vi "DataTreeCtrl signalToIonData.vi"(8 "error in (no error)":errorcluster, 10 "signalData":waveform(sgl), 11 "DataTreeCtrl in":refnum<class "DataTreeCtrl.lvclass">) -> (0 "error out":errorcluster, 2 "ionSigInfo":T1, 3 "DataTreeCtrl out":refnum<class "DataTreeCtrl.lvclass">, 5 "plotName":string)   [LabVIEW 2018, in "DataTreeCtrl.lvclass"]
uses:
  DataTreeCtrl.lvclass
  DataTreeCtrl.lvclass/DataTreeCtrl.ctl
  PublicSubVI/Class/Sig2MS/Sig2MS.lvclass
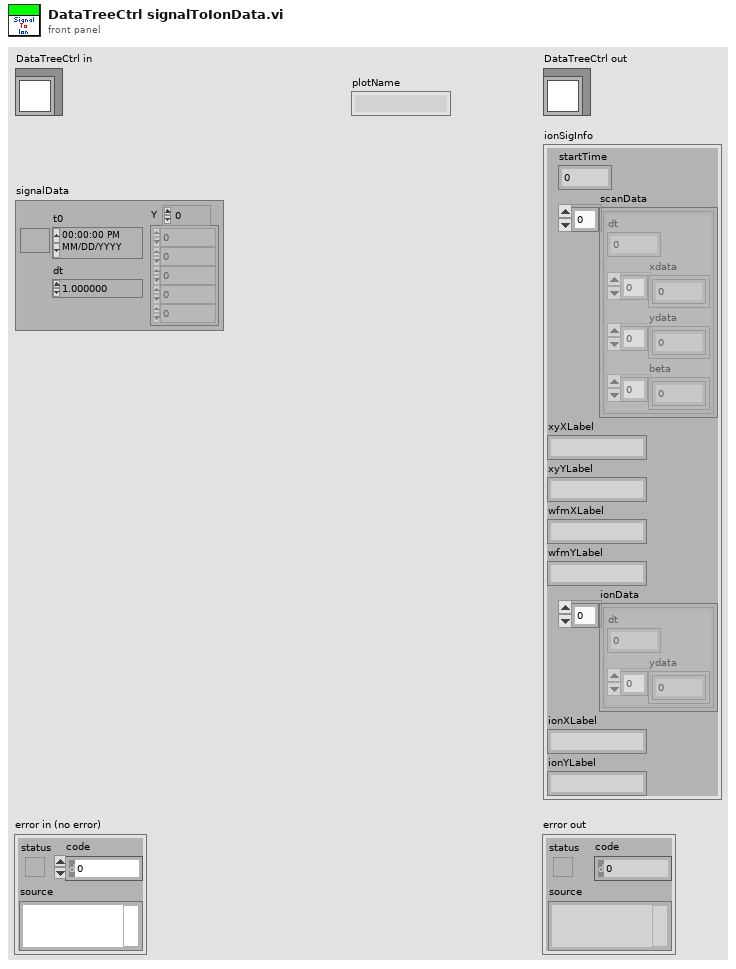
[diagram p1: front panel]
types:
  T1 = cluster{"startTime":dbl, "scanData":cluster{"dt":dbl, "xdata":dbl[], "ydata":sgl[], "beta":dbl[]}[], "xyXLabel":string, "xyYLabel":string, "wfmXLabel":string, "wfmYLabel":string, "ionData":cluster{"dt":dbl, "ydata":sgl[]}[], "ionXLabel":string, "ionYLabel":string}
  T2 = enum16{"init", "loadScript", "newScript", "runScript", "close"}
  T3 = cluster{"startTime":dbl, "scanSig":cluster{"priDt":dbl, "priXData":dbl[], "priYData":sgl[], "beta":dbl[]}[], "ionSig":cluster{"secDt":dbl, "secYData":sgl[]}[]}
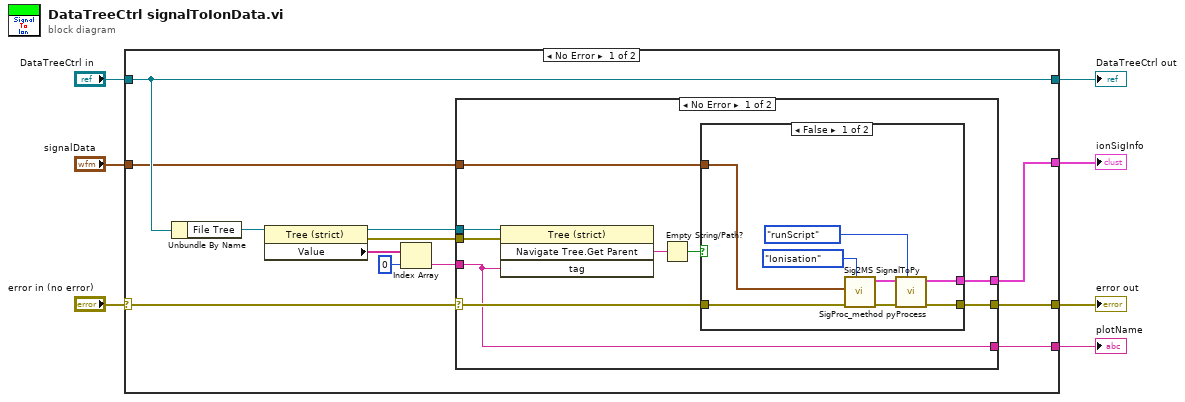
[diagram p0: block diagram]
diagram:
  n1 = case shown="No Error" "error in (no error)" {
    selector: "error in (no error)" -> [w15 w40]
    tunnel: [w14 w40] -> w4
    tunnel: [w19 w39] -> w5
    tunnel: "DataTreeCtrl in" -> [w19 w39]
    tunnel: "signalData" -> [w13 _]
    tunnel: [w9 _] -> w2
    tunnel: [w8 _] -> w1
    frame No Error {
      n2 = Unbundle By Name(w19) -> ("File Tree"=w18:refnum<vi>)
      n3 = property class="Tree (strict)"(reference=w18) -> (reference out=w17:refnum<vi>, error out=w16:errorcluster, "Value"=w12:string[])  [unwired: 1 in]
      n4 = Index Array(array=w12, index=0) -> (element=w10:string)
      n5 = case shown="No Error" w15 {
        selector: w15 -> [w23 w38]
        tunnel: w17 -> [w28 _]
        tunnel: w16 -> [w27 _]
        tunnel: [w24 w38] -> w14
        tunnel: w13 -> [w22 _]
        tunnel: w10 -> [w21 _]
        tunnel: [w21 _] -> w9
        tunnel: [w20 _] -> w8
        frame No Error {
          n6 = invoke class="Tree (strict)" method="Navigate Tree.Get Parent"(reference=w28, error in=w27, "tag"=w21) -> ("Navigate Tree:Get Parent"=w25:string)  [unwired: 1 in, 3 out]
          n7 = Empty String/Path?(string/path=w25) -> (empty?=w26:bool)
          n8 = case shown="False" w26 {
            tunnel: [w30 w37] -> w24
            tunnel: w23 -> [w32 w37]
            tunnel: w22 -> [w33 _]
            tunnel: [w31 _] -> w20
            frame False {
              n9 = call "Sig2MS SignalToPy.vi"("getType"=enum16{"All", "Spectra", "Ionisation"}."Ionisation", "error in (no error)"=w32, "rawSignal"=w33) -> ("error out"=w35:errorcluster, "pySigFormat"=w36:T3)  [unwired: 7 in]
              n10 = call "SigProc_method pyProcess.vi"("func"=T2."runScript", "error in (no error)"=w35, "dataParam"=w36) -> ("error out"=w30:errorcluster, "newSigInfo"=w31:T1)  [unwired: 5 in, 2 out]
            }
            frame True {
            }
          }
        }
        frame Error {
        }
      }
    }
    frame Error {
    }
  }
  "error out" <- w4
  "DataTreeCtrl out" <- w5
  "plotName" <- w2
  "ionSigInfo" <- w1
